vi "Simple Rendezvous.vi"() -> ()   [LabVIEW 2023]
doc: "This VI creates a rendezvous and calls two parallel loops that will use the rendezvous to synchronize the start of their updates. A rendezvous is most useful when you have parallel processes that may take different amounts of time to execute, but must always start at the same time."
panel:
  out "Total 2":i32
  out "Total 1":i32
  out "Waiting for Loop 1?":bool
  out "Waiting for Loop 2?":bool
  out "Data 2":i32(graph)
  out "Data 1":i32(graph)
  in  "Stop":bool
  # "Overview: Demonstrates the use of the Rendezvous VIs to synchronize the start of execution of parallel code.\nInstructions:\nRun the VI."
  # "The Data charts will always start updating at the same time. One will finish before the other. The second chart must finish updating before both charts start again."
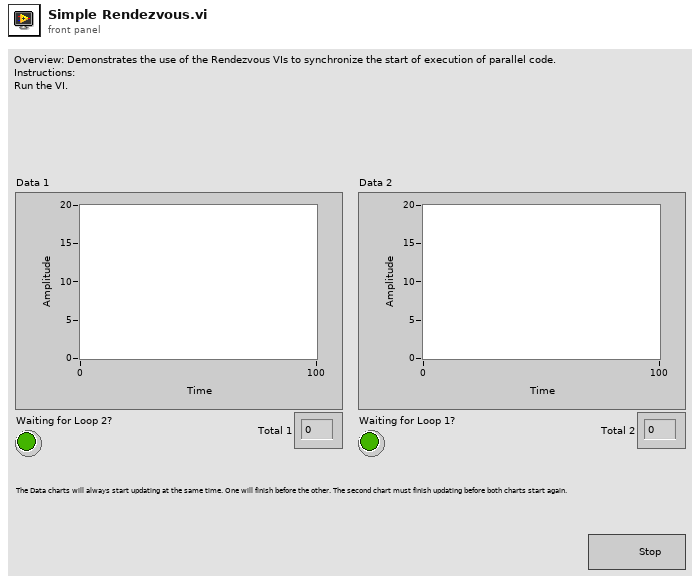
[diagram p1: front panel]
types:
  T1 = typedef "Rendezvous RefNum" = refnum<k1>
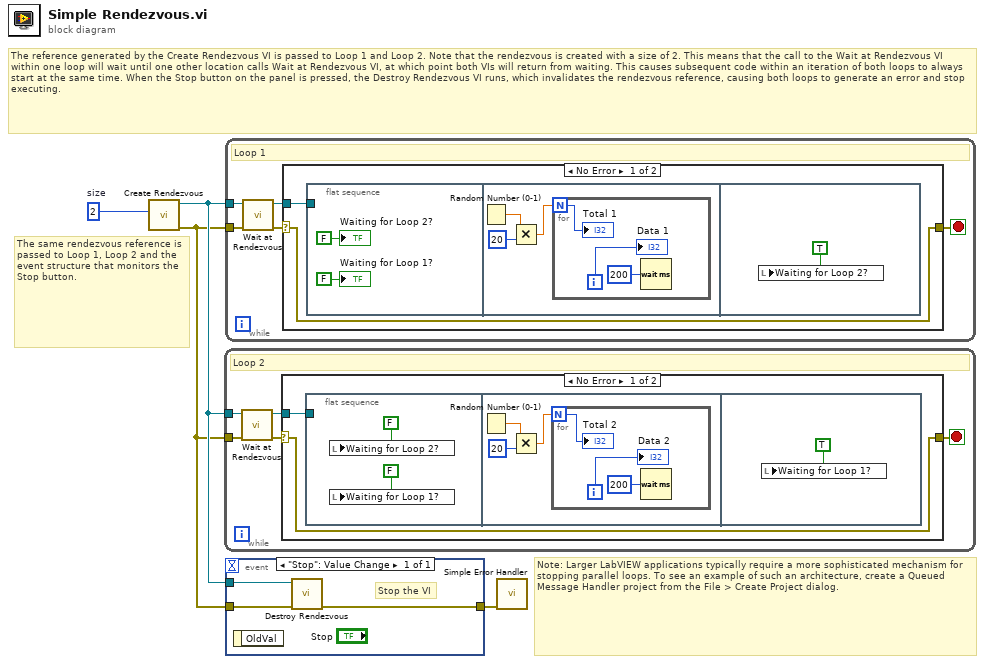
[diagram p0: block diagram]
diagram:
  w1 = 2  # size
  # "Note: Larger LabVIEW applications typically require a more sophisticated mechanism for stopping parallel loops. To see an example of such an architecture, create a Queued Message Handler project from the File > Create Project dialog."
  # "The same rendezvous reference is passed to Loop 1, Loop 2 and the event structure that monitors the Stop button."
  # "The reference generated by the Create Rendezvous VI is passed to Loop 1 and Loop 2. Note that the rendezvous is created with a size of 2. This means that the call to the Wait at Rendezvous VI within one loop will wait until one other location calls Wait at Rendezvous VI, at which point both VIs will return from waiting. This causes subsequent code within an iteration of both loops to always start at the same time. When the Stop button on the panel is pressed, the Destroy Rendezvous VI runs, which invalidates the rendezvous reference, causing both loops to generate an error and stop executing."
  n1 = call <vilib>:"Create Rendezvous.vi"("size (2)"=w1) -> ("error out"=w2:errorcluster, "rendezvous"=w3:T1)  [unwired: 4 in, 1 out]
  n2 = while {
    tunnel: w3 -> [w9]
    tunnel: w2 -> [w8]
    stop <- w6 stop-if-true
    # "Loop 2"
    n3 = call <vilib>:"Wait at Rendezvous.vi"("error in (no error)"=w8, "rendezvous"=w9) -> ("error out"=w5:errorcluster, "rendezvous out"=w7:T1)  [unwired: 3 in, 1 out]
    n4 = case shown="No Error" w5 {
      selector: w5 -> [w10 w21]
      tunnel: w7 -> [w11 _]
      tunnel: [w10 w21] -> w6
      frame No Error {
        n5 = flat-sequence {
          tunnel: w11 -> [_]
          frame #0 {
            n6 = local write "Waiting for Loop 2?"(FALSE ("Loop 1 Access?")) -> ()
            n7 = local write "Waiting for Loop 1?"(FALSE ("Loop 2 Access?")) -> ()
          }
          frame #1 {
            n8 = Random Number (0-1)() -> (number: 0 to 1=w16:dbl)
            n9 = Multiply(x=w16, y=20) -> (x*y=w15:dbl)
            n10 = for {
              N: w15 -> [w17]
              i -> [w18]
              n11 = Wait (ms)(milliseconds to wait=u32 200) -> ()  [unwired: 1 out]
              "Data 2" <- w18
              "Total 2" <- w17
            }
          }
          frame #2 {
            n12 = local write "Waiting for Loop 1?"(TRUE ("Loop 2 Access?")) -> ()
          }
        }
      }
      frame Error {
        # "Rendezvous reference was closed. Stop loop."
      }
    }
  }
  n13 = while {
    tunnel: w3 -> [w26]
    tunnel: w2 -> [w25]
    stop <- w23 stop-if-true
    # "Loop 1"
    n14 = call <vilib>:"Wait at Rendezvous.vi"("error in (no error)"=w25, "rendezvous"=w26) -> ("error out"=w22:errorcluster, "rendezvous out"=w24:T1)  [unwired: 3 in, 1 out]
    n15 = case shown="No Error" w22 {
      selector: w22 -> [w27 w38]
      tunnel: w24 -> [w28 _]
      tunnel: [w27 w38] -> w23
      frame No Error {
        n16 = flat-sequence {
          tunnel: w28 -> [_]
          frame #0 {
            "Waiting for Loop 2?" <- FALSE ("Loop 1 Access?")
            "Waiting for Loop 1?" <- FALSE ("Loop 2 Access?")
          }
          frame #1 {
            n17 = Random Number (0-1)() -> (number: 0 to 1=w31:dbl)
            n18 = Multiply(x=w31, y=20) -> (x*y=w32:dbl)
            n19 = for {
              N: w32 -> [w34]
              i -> [w35]
              n20 = Wait (ms)(milliseconds to wait=u32 200) -> ()  [unwired: 1 out]
              "Data 1" <- w35
              "Total 1" <- w34
            }
          }
          frame #2 {
            n21 = local write "Waiting for Loop 2?"(TRUE ("Loop 1 Access?")) -> ()
          }
        }
      }
      frame Error {
        # "Rendezvous reference was closed. Stop loop."
      }
    }
  }
  n22 = event shown="[0] \"Stop\": Value Change" {
    selector: _ -> [_]
    dyn-events: _ -> [_]
    timeout: _ -> [_]
    tunnel: w2 -> [w40]
    tunnel: w3 -> [w41]
    tunnel: [w39] -> w4
    event "Stop": Value Change {
      # "Stop the VI"
      n23 = event-data() -> ()  [unwired: 1 in, 1 out]
      n24 = call <vilib>:"Destroy Rendezvous.vi"("error in (no error)"=w40, "rendezvous"=w41) -> ("error out"=w39:errorcluster)  [unwired: 4 in, 1 out]
    }
  }
  n25 = call <vilib>:"Simple Error Handler.vi"("error in (no error)"=w4) -> ()  [unwired: 4 in, 5 out]
